vi "PADMINI FALSE TRUE TO STRING.vi"(10 "RESULT":bool) -> (2 "RESULT":string)   [LabVIEW 2017]
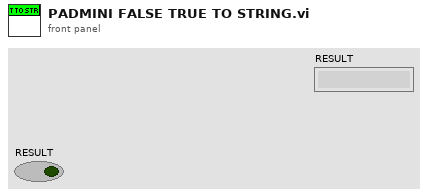
[diagram p1: front panel]
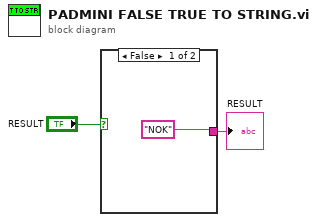
[diagram p0: block diagram]
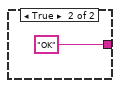
[diagram p2: hidden frame]
diagram:
  n1 = case shown="False" "RESULT" {
    tunnel: ["NOK" "OK"] -> w1
    frame False {
    }
    frame True {
    }
  }
  "RESULT" <- w1
